vi "GUI Wavefrom Panel.vi"(8 "error in":errorcluster, 11 "source name":string="last record") -> (0 "error out":errorcluster)   [LabVIEW 2013]
doc: "Viewer of the record waveforms."
uses:
  GUI Waveform Info.ctl
panel:
  in  "avg index":u16(ring) caption="Average index" items=["Last", "Cycle 0", "Cycle 1", "Cycle 2"]
  in  "grp index":u16(ring) caption="Group index" items=["Last", "Group 0"]
  out "Current record path":path
  in  "max smpl":i32=1000 caption="Max samples to display"
  in  "first smpl [%]":dbl(slide) caption="First sample to display [%]" min=0.0 max=100.0 step=0.1 scale=0.0..100.0
  out "Channel waveforms":T1(graph)
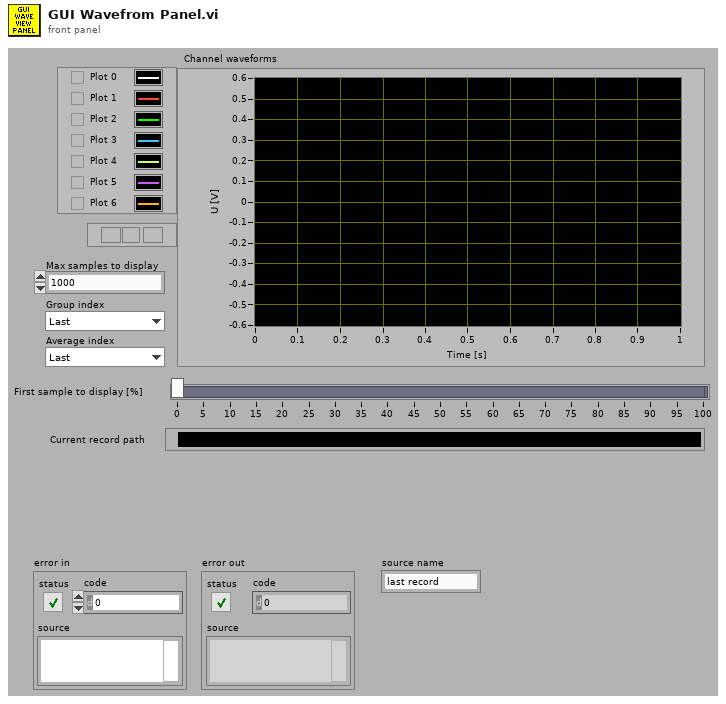
[diagram p1: front panel]
types:
  T1 = cluster{"time [s]":ext[], "waveforms [V]":sgl[]}[]
  T2 = typedef "GUI Waveform Info.ctl" = cluster{"header path":path, "group id":i32, "average id":i32, "Time Stamp":timestamp, "max samples":i64, "first sample":i64, "first smpl [%]":dbl}
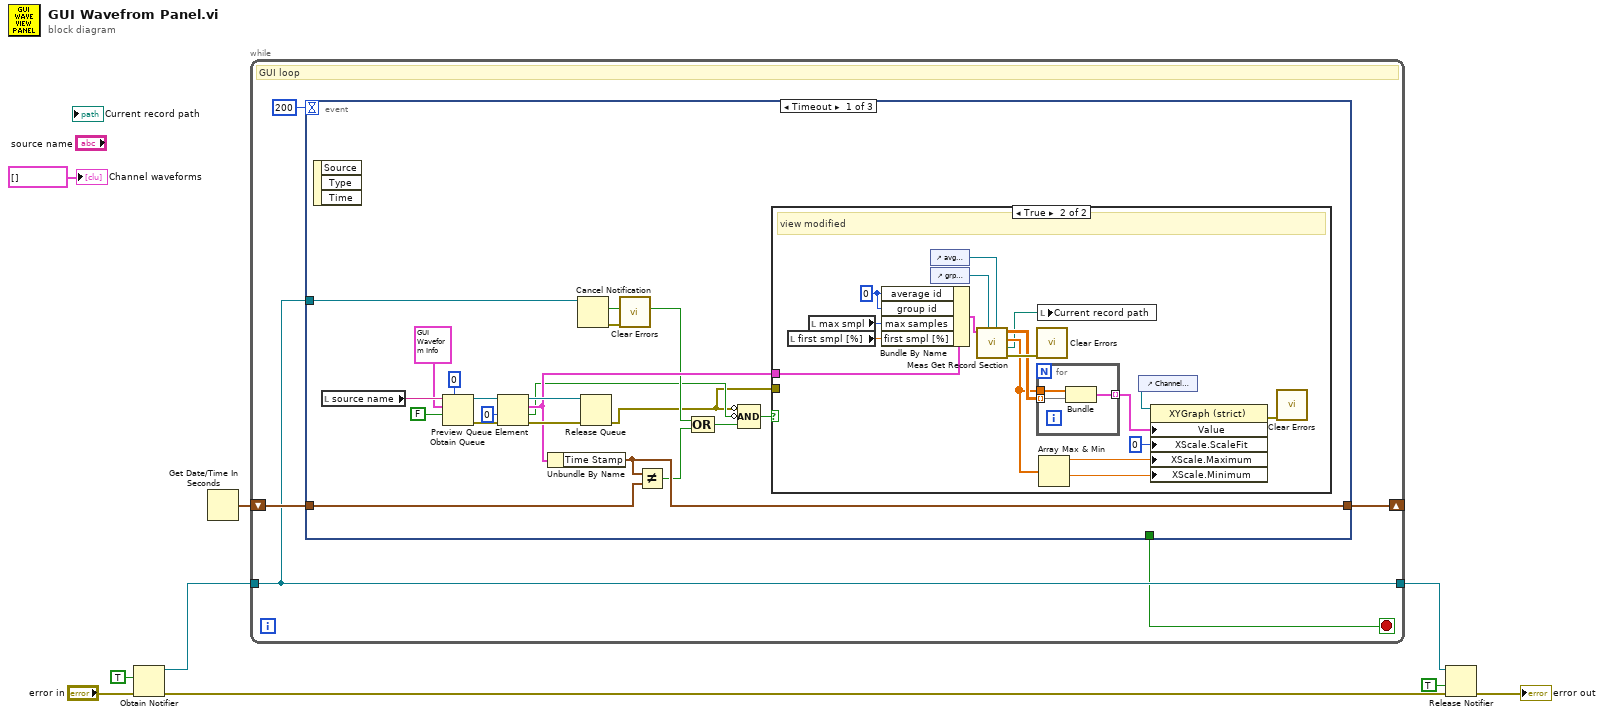
[diagram p0: block diagram]
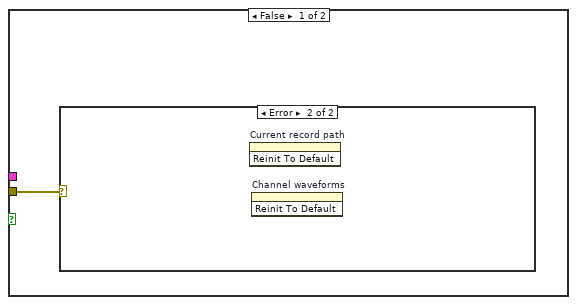
[diagram p2: hidden frame]
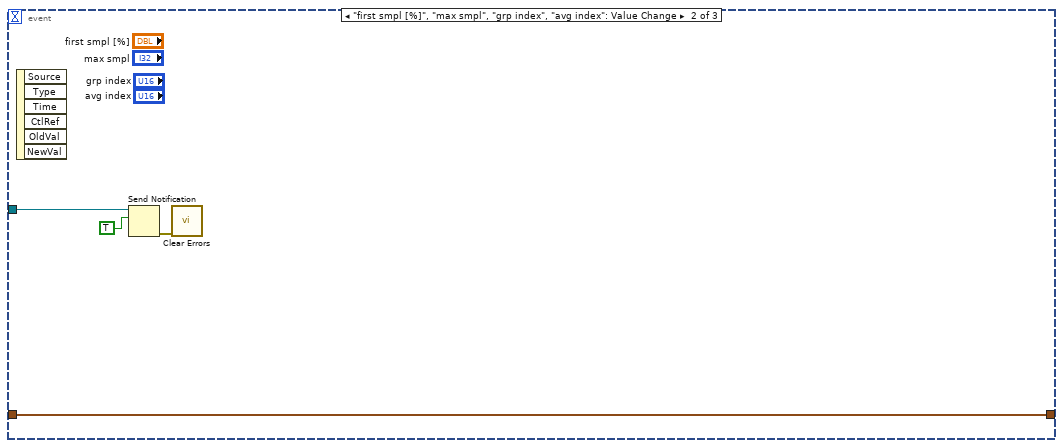
[diagram p4: hidden frame]
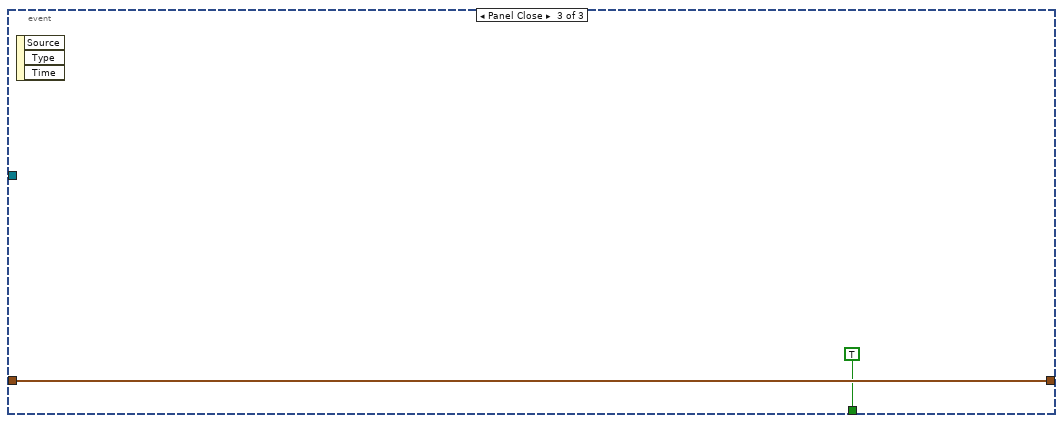
[diagram p5: hidden frame]
diagram:
  n1 = Obtain Notifier(notification data type=TRUE, error in (no error)="error in") -> (notifier out=w2:refnum<notifier>, error out=w6:errorcluster)  [unwired: 2 in, 1 out]
  n2 = Get Date/Time In Seconds() -> (seconds since 1Jan1904=w9:timestamp)
  n3 = while {
    shift-right: [w12] -> _
    shift-left: w9 -> [w13]
    tunnel: [w11] -> w3
    tunnel: w2 -> [w11]
    stop <- w10 stop-if-true
    # "GUI loop"
    n4 = event shown="[0] Timeout" {
      selector: _ -> [_ _ _]
      dyn-events: _ -> [_ _ _]
      timeout: 200 -> [_ _ _]
      tunnel: w13 -> [w26 w59 w61]
      tunnel: [w25 w59 w61] -> w12
      tunnel: w11 -> [w23 w58 _]
      tunnel: [_ _ TRUE] -> w10
      event Timeout {
        n5 = event-data() -> ()  [unwired: 1 in, 3 out]
        n6 = local read "source name"() -> (w34:string)
        n7 = Obtain Queue(max queue size (-1, unlimited)=0, name (unnamed)=w34, element data type=T2 {"header path"=path "", "group id"=0, "average id"=0, "Time Stamp"=timestamp(0 s since 1904-01-01), "max samples"=0, "first sample"=0, "first smpl [%]"=0.0} ("record info"), create if not found? (T)=FALSE) -> (queue out=w31:refnum<queue>, error out=w16:errorcluster)  [unwired: 1 in, 1 out]
        n8 = Preview Queue Element(queue=w31, timeout in ms (-1)=0, error in (no error)=w16) -> (queue out=w30:refnum<queue>, element=w24:T2, timed out?=w17:bool, error out=w32:errorcluster)
        n9 = Unbundle By Name(w24) -> ("Time Stamp"=w25:timestamp)
        n10 = Cancel Notification(0:w23) -> (9:w21:bool, 11:w20:errorcluster)  [unwired: 1 in, 1 out]
        n11 = Release Queue(queue=w30, error in (no error)=w32) -> (error out=w15:errorcluster)  [unwired: 1 in, 2 out]
        n12 = call <vilib>:"Clear Errors.vi"("error in (no error)"=w20) -> ()  [unwired: 6 in, 1 out]
        n13 = Not Equal?(x=w25, y=w26) -> (x != y?=w22:bool)
        n14 = Compound Arithmetic op=OR(w21, w22) -> (w19:bool)
        n15 = Compound Arithmetic op=AND(invert w15, invert w17, w19) -> (w18:bool)
        n16 = case shown="True" w18 {
          tunnel: w24 -> [_ w52]
          tunnel: w15 -> [w35 _]
          frame False {
            n17 = case shown="Error" w35 {
              frame No Error {
              }
              frame Error {
                n18 = invoke on="Current record path" class="Path" method="Reinit To Default"() -> ()  [unwired: 3 in, 3 out]
                n19 = invoke on="Channel waveforms" class="XYGraph (strict)" method="Reinit To Default"() -> ()  [unwired: 3 in, 3 out]
              }
            }
          }
          frame True {
            w38 = 0 ("average id")
            # "view modified"
            n20 = local read "first smpl [%]"() -> (w50:dbl)
            n21 = local read "max smpl"() -> (w51:i32)
            n22 = Bundle By Name(cluster=w52, "average id"=w38, "group id"=w38, "max samples"=w51, "first smpl [%]"=w50) -> (w49:T2)
            n23 = control-ref of="avg index"() -> (w36:refnum<vi>)
            n24 = control-ref of="grp index"() -> (w37:refnum<vi>)
            n25 = call "Meas Get Record Section.vi"("avg index ref"=w36, "grp index ref"=w37, "record info"=w49) -> ("error out"=w48:errorcluster, "record path"=w39:path, "time [s]"=w45:ext[], "waveforms [V]"=w47:sgl[][])  [unwired: 5 in]
            n26 = call <vilib>:"Clear Errors.vi"("error in (no error)"=w48) -> ()  [unwired: 6 in, 1 out]
            n27 = for {
              tunnel: w47 -> [w55] mode=indexing
              tunnel: w45 -> [w54]
              tunnel: [w53] -> w41 mode=indexing
              n28 = Bundle("time [s]"=w54, "waveforms [V]"=w55) -> (w53:cluster{"time [s]":ext[], "waveforms [V]":sgl[]})  [unwired: 1 in]
            }
            n29 = local write "Current record path"(w39) -> ()
            n30 = Array Max & Min(array=w45) -> (max value=w44:ext, min value=w43:ext)  [unwired: 2 out]
            n31 = control-ref of="Channel waveforms"() -> (w46:refnum<vi>)
            n32 = property class="XYGraph (strict)"(reference=w46, "Value"=w41, "XScale.ScaleFit"=u8 0 ("X Scale.Scale Fit"), "XScale.Maximum"=w44, "XScale.Minimum"=w43) -> (error out=w42:errorcluster)  [unwired: 1 in, 1 out]
            n33 = call <vilib>:"Clear Errors.vi"("error in (no error)"=w42) -> ()  [unwired: 6 in, 1 out]
          }
        }
      }
      event "first smpl [%]", "max smpl", "grp index", "avg index": Value Change {
        n34 = event-data() -> ()  [unwired: 1 in, 6 out]
        n35 = Send Notification(notification=TRUE, notifier=w58) -> (error out=w56:errorcluster)  [unwired: 1 in, 1 out]
        n36 = call <vilib>:"Clear Errors.vi"("error in (no error)"=w56) -> ()  [unwired: 6 in, 1 out]
      }
      event Panel Close {
        n37 = event-data() -> ()  [unwired: 1 in, 3 out]
      }
    }
  }
  n38 = Release Notifier(notifier=w3, force destroy? (F)=TRUE, error in (no error)=w6) -> (error out=→"error out":errorcluster)  [unwired: 2 out]
  "Channel waveforms" <- T1 [] ("XY Graph")
